vi "Format Page Header.vi"(6 "Library Scope":T1(ring), 9 "Description":string, 10 "Qualified Name":string, 11 "Name":string) -> (3 "Text Output":string)   [LabVIEW 2023, in "VIDoc Printer - Confluence.lvlib" / "VIDoc Printer - Confluence.lvclass"]
uses:
  VIDoc Printer - Confluence.lvclass
  Confluence Formatting/Types/Format Combo Box.ctl
  Confluence Formatting/Layout - Two.vi
  VIDoc Printer - Confluence.lvclass/VIDoc Printer - Confluence.ctl
  Confluence Formatting/Confluence Formatting.lvlib
  <userlib>/_PetranWay/LabVIEW Confluence API/Source/PetranWay_Confluence API.lvlib
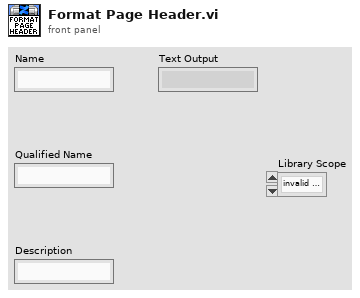
[diagram p1: front panel]
types:
  T1 = enum32{"invalid scope", "public", "private", "protected", "community"}
  T2 = typedef "Confluence Formatting.lvlib/Format Combo Box.ctl" = string
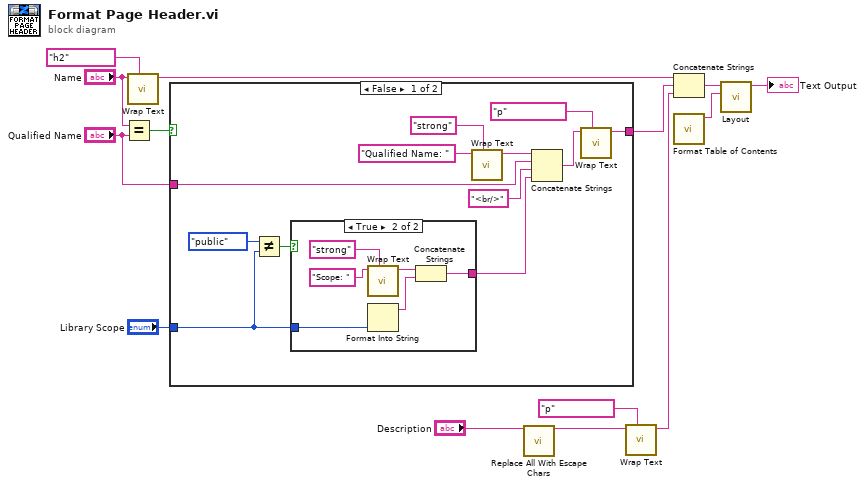
[diagram p0: block diagram]
diagram:
  n1 = Equal?(x="Name", y="Qualified Name") -> (x = y?=w3:bool)
  n2 = call "Wrap Text.vi"("Formatting"=T2 "h2", "String"="Name") -> ("Wrapped String"=w7:string)  [unwired: 8 in, 1 out]
  n3 = case shown="False" w3 {
    tunnel: [w26 _] -> w14
    tunnel: "Qualified Name" -> [w22 _]
    tunnel: "Library Scope" -> [w16 _]
    frame False {
      n4 = Not Equal?(x=T1."public" ("y"), y=w16) -> (x != y?=w17:bool)
      n5 = case shown="True" w17 {
        tunnel: w16 -> [_ w30]
        tunnel: [_ w27] -> w15
        frame False {
        }
        frame True {
          n6 = call "Wrap Text.vi"("Formatting"=T2 "strong", "String"="Scope: ") -> ("Wrapped String"=w31:string)  [unwired: 8 in, 1 out]
          n7 = Format Into String(w30) -> (resulting string=w29:string)  [unwired: 3 in, 1 out]
          n8 = Concatenate Strings(w31, w29) -> (w27:string)
        }
      }
      n9 = call "Wrap Text.vi"("Formatting"=T2 "strong", "String"="Qualified Name: " ("string")) -> ("Wrapped String"=w23:string)  [unwired: 8 in, 1 out]
      n10 = Concatenate Strings(w23, w22, "<br/>" ("string"), w15) -> (w21:string)
      n11 = call "Wrap Text.vi"("Formatting"=T2 "p", "String"=w21) -> ("Wrapped String"=w26:string)  [unwired: 8 in, 1 out]
    }
    frame True {
    }
  }
  n12 = call <userlib>:"Replace All With Escape Chars.vi"("Raw String"="Description") -> ("With Substitued Escape Characters"=w1:string)  [unwired: 13 in, 1 out]
  n13 = call "Wrap Text.vi"("Formatting"=T2 "p", "String"=w1) -> ("Wrapped String"=w8:string)  [unwired: 8 in, 1 out]
  n14 = Concatenate Strings(w7, w14, w8) -> (w10:string)
  n15 = call "Format Table of Contents.vi"() -> ("Table of Contents String"=w9:string)  [unwired: 10 in, 1 out]
  n16 = call-poly "Layout.vi"("Section 2"=w9, "Section 1"=w10) -> ("Text Output"=→"Text Output":string)  [unwired: 8 in, 1 out]
